vi "Test JSON to Variant 2.vi"() -> ()   [LabVIEW 2011]
uses:
  JSON Value/Set from JSON string.vi
  JSON Value/Get as JSON string (pretty).vi
  JSON Value/JSON Value.lvclass
  Variant JSON.lvlib
  Get Polymorphic/JSON GetSet.lvlib
panel:
  out "Variant after setting":variant
  out "Cluster after setting":T1
  in  "Cluster to set":T2
  in  "Creation cluster":T3={"T2"="Test \"quote\",\nand newline.", "Nest"={"Enum"=enum."CCC", "NestNest"={"A"=34.0, "Complex"=2.0+3.1i, "C"="1.23 string"}}, "Test Array"=[456.789, 2.0, 3.0], "Boolean 1"=TRUE, "T1"=456.789, "Boolean 2"="true (a string)", "Time Stamp"=timestamp(3434102896.3125 s since 1904-01-01), "Extra item"="test2", "Non JSON valid numerics"=inf, "NAN"=nan, "TTT"="", "signal in"={"t0"=timestamp(3436250625 s since 1904-01-01), "dt"=1.0, "Y"=[23.0, 34.0]}, "Path"=path ""}
  out "JSON String created":string
  # "see diagram"
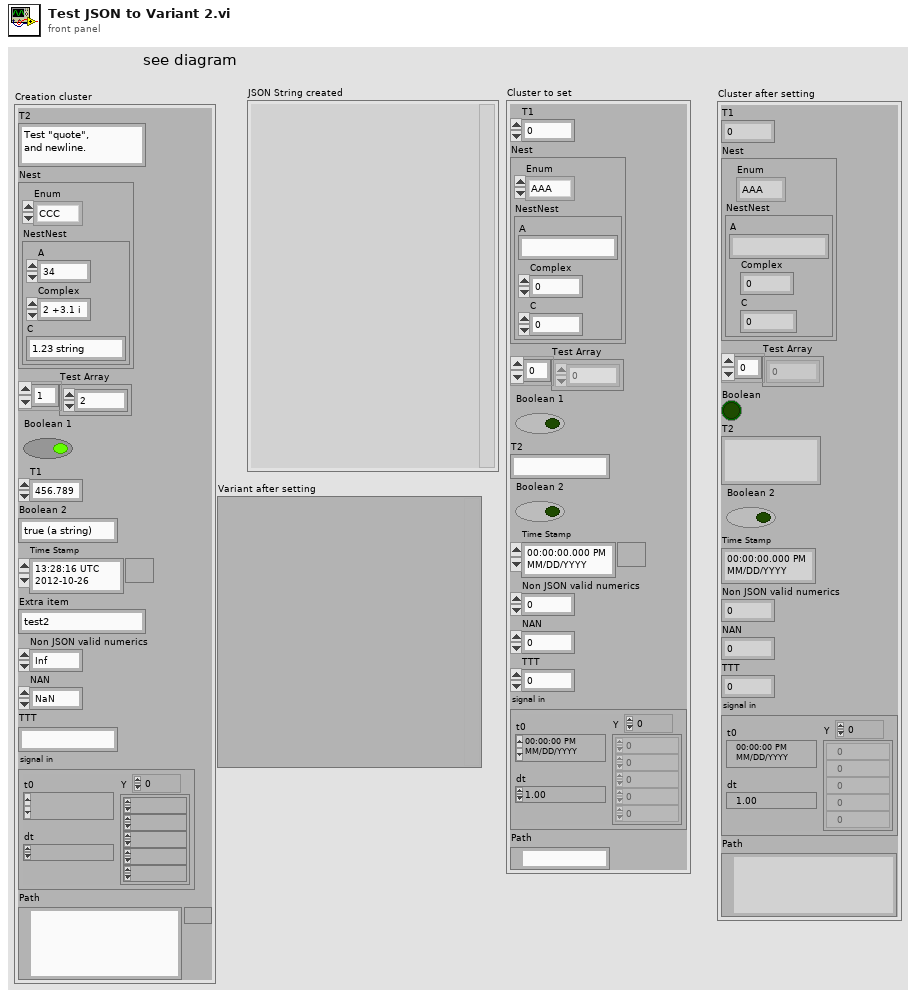
[diagram p1: front panel]
types:
  T1 = cluster{"T1":dbl, "Nest":cluster{"Enum":enum16{"AAA", "BBB", "CCC"}, "NestNest":cluster{"A":string, "Complex":cdb, "C":dbl}}, "Test Array":dbl[], "Boolean":bool, "T2":string, "Boolean 2":bool, "Time Stamp":timestamp, "Non JSON valid numerics":dbl, "NAN":dbl, "TTT":dbl, "signal in":waveform(dbl), "Path":path}
  T2 = cluster{"T1":dbl, "Nest":cluster{"Enum":enum16{"AAA", "BBB", "CCC"}, "NestNest":cluster{"A":string, "Complex":cdb, "C":dbl}}, "Test Array":dbl[], "Boolean 1":bool, "T2":string, "Boolean 2":bool, "Time Stamp":timestamp, "Non JSON valid numerics":dbl, "NAN":dbl, "TTT":dbl, "signal in":waveform(dbl), "Path":path}
  T3 = cluster{"T2":string, "Nest":cluster{"Enum":enum16{"AAA", "BBB", "CCC"}, "NestNest":cluster{"A":dbl, "Complex":cdb, "C":string}}, "Test Array":dbl[], "Boolean 1":bool, "T1":dbl, "Boolean 2":string, "Time Stamp":timestamp, "Extra item":string, "Non JSON valid numerics":dbl, "NAN":dbl, "TTT":string, "signal in":waveform(dbl), "Path":path}
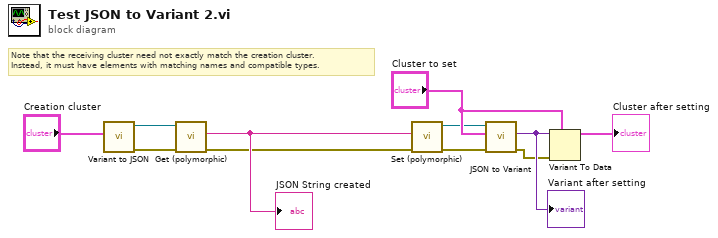
[diagram p0: block diagram]
diagram:
  # "Note that the receiving cluster need not exactly match the creation cluster.\nInstead, it must have elements with matching names and compatible types."
  n1 = call "Variant to JSON.vi"("Variant"="Creation cluster") -> ("error out"=w4:errorcluster, "JSON Value out"=w11:refnum<class "JSON Value.lvclass">)  [unwired: 9 in]
  n2 = call-poly "Get (polymorphic).vi"("error in (no error)"=w4, "JSON Value in"=w11) -> ("error out"=w3:errorcluster, "String"=w5:string)  [unwired: 8 in]
  "JSON String created" <- w5
  n3 = call-poly "Set (polymorphic).vi"("error in (no error)"=w3, "JSON stream"=w5) -> ("error out"=w1:errorcluster, "JSON Value out"=w2:refnum<class "JSON Value.lvclass">)  [unwired: 7 in, 1 out]
  n4 = call "JSON to Variant.vi"("error in (no error)"=w1, "Variant (Data Type)"="Cluster to set", "JSON Value"=w2) -> ("error out"=w7:errorcluster, "Variant out"=w10:variant)  [unwired: 7 in]
  "Variant after setting" <- w10
  n5 = Variant To Data(error in=w7, type="Cluster to set", Variant=w10) -> (data=→"Cluster after setting":T2)  [unwired: 1 out]
